vi "Reset Voltages.vi"(7 "index":i32, 8 "error in (no error)":errorcluster, 9 "WL Voltage (V)":dbl, 10 "SL Voltage (V)":dbl, 11 "IVI Refnum in":refnum<k15>) -> (0 "error out":errorcluster, 3 "IVI Refnum out":refnum<k15>)   [LabVIEW 2018]
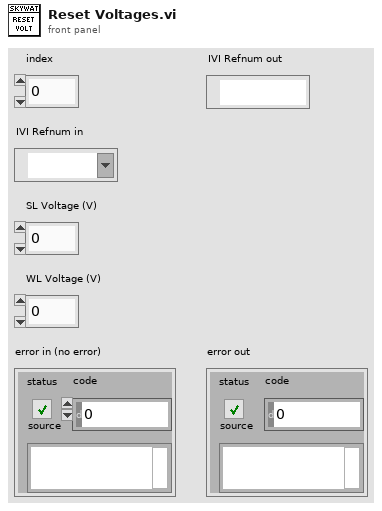
[diagram p1: front panel]
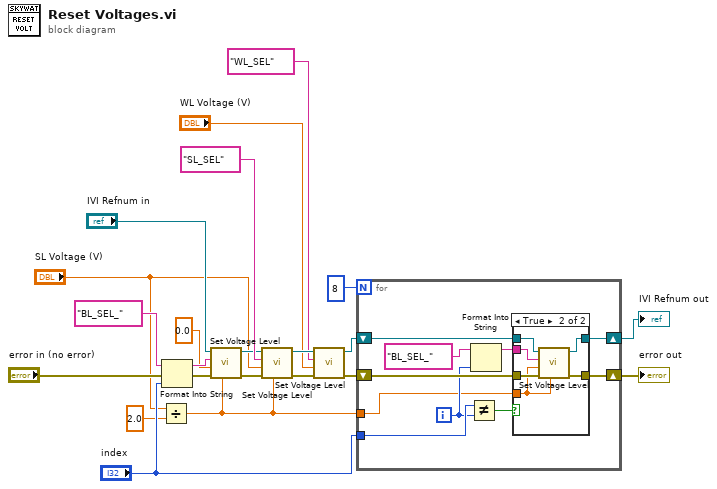
[diagram p0: block diagram]
diagram:
  n1 = Divide(x="SL Voltage (V)", y=2.0) -> (x/y=w1:dbl)
  n2 = Format Into String(initial string="BL_SEL_" ("channel list"), error in="error in (no error)", "index") -> (resulting string=w22:string, error out=w20:errorcluster)  [unwired: 1 in]
  n3 = call "Set Voltage Level.vi"("low level"=w1, "error in (no error)"=w20, "level (V)"=0.0, "channel list"=w22, "instrument handle"="IVI Refnum in") -> ("error out"=w16:errorcluster, "instrument handle out"=w17:refnum<k15>)  [unwired: 5 in]
  n4 = call "Set Voltage Level.vi"("low level"=w1, "error in (no error)"=w16, "level (V)"="SL Voltage (V)", "channel list"="SL_SEL", "instrument handle"=w17) -> ("error out"=w3:errorcluster, "instrument handle out"=w8:refnum<k15>)  [unwired: 5 in]
  n5 = call "Set Voltage Level.vi"("error in (no error)"=w3, "level (V)"="WL Voltage (V)", "channel list"="WL_SEL", "instrument handle"=w8) -> ("error out"=w6:errorcluster, "instrument handle out"=w7:refnum<k15>)  [unwired: 6 in]
  n6 = for {
    N: 8 -> [_]
    tunnel: "index" -> [w32]
    shift-right: [w30] -> w12
    shift-left: w7 -> [w31]
    shift-right: [w28] -> w11
    shift-left: w6 -> [w29]
    tunnel: w1 -> [w23]
    i -> [w26]
    n7 = Not Equal?(x=w32, y=w26) -> (x != y?=w27:bool)
    n8 = Format Into String(initial string="BL_SEL_" ("channel list"), w26) -> (resulting string=w24:string)  [unwired: 2 in, 1 out]
    n9 = case shown="True" w27 {
      tunnel: w31 -> [w34 w40]
      tunnel: [w34 w39] -> w30
      tunnel: w29 -> [w33 w38]
      tunnel: [w33 w37] -> w28
      tunnel: w24 -> [_ w36]
      tunnel: w23 -> [_ w35]
      frame False {
      }
      frame True {
        n10 = call "Set Voltage Level.vi"("low level"=w35, "error in (no error)"=w38, "level (V)"=w35, "channel list"=w36, "instrument handle"=w40) -> ("error out"=w37:errorcluster, "instrument handle out"=w39:refnum<k15>)  [unwired: 5 in]
      }
    }
  }
  "IVI Refnum out" <- w12
  "error out" <- w11
